vi "float_add.vi"(11 "x":sgl) -> (3 "y":sgl)   [LabVIEW 2018, in "posit.lvlib"]
uses:
  posit.lvlib
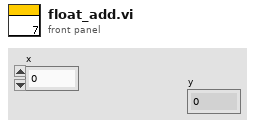
[diagram p1: front panel]
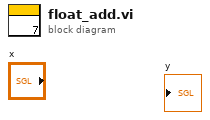
[diagram p0: block diagram]
diagram:
